vi "Get Daemon Error.vi"(8 "Error In":errorcluster, 11 "Error Reference":refnum<data-value>) -> (0 "Error Out":errorcluster)   [LabVIEW 2019, in "TDMS Logger.lvlib" / "TDMS Logger.lvclass"]
uses:
  TDMS Logger.lvclass
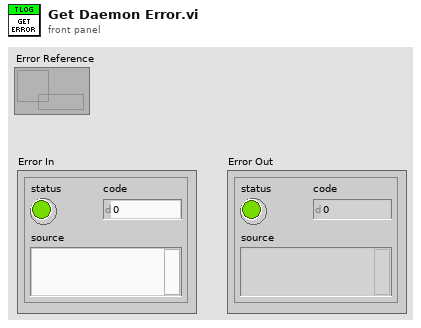
[diagram p1: front panel]
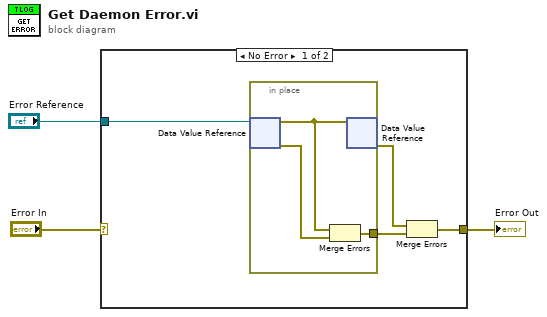
[diagram p0: block diagram]
diagram:
  n1 = case shown="No Error" "Error In" {
    selector: "Error In" -> [_ w11]
    tunnel: [w5 w11] -> w2
    tunnel: "Error Reference" -> [w4 _]
    frame No Error {
      n2 = in-place {
        in-place-border: [w8] -> w7
        n3 = in-place-dvr #1(w4) -> (w9:errorcluster, w10:errorcluster)
        n4 = Merge Errors(w9, w10) -> (w8:errorcluster)
        n5 = in-place-dvr #1(w9) -> (w6:errorcluster)  [unwired: 1 out]
      }
      n6 = Merge Errors(w6, w7) -> (w5:errorcluster)
    }
    frame Error {
    }
  }
  "Error Out" <- w2
